vi "Make 16 to 8 LUT.vi"(1 "Black level":dbl format="%.2f", 2 "White level":dbl format="%.2f") -> (0 "Lookup Table":i16[](array[numeric]))   [LabVIEW 2011]
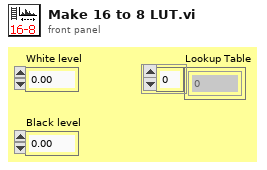
[diagram p1: front panel]
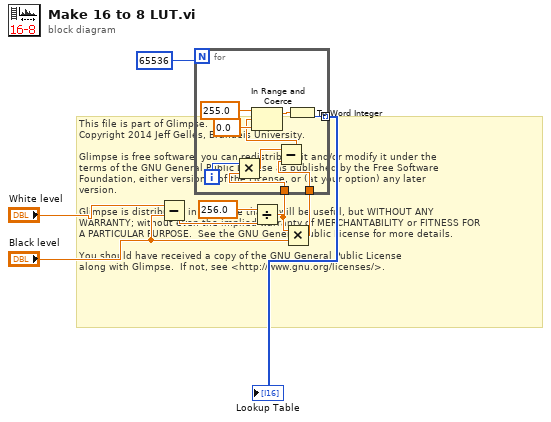
[diagram p0: block diagram]
diagram:
  # "This file is part of Glimpse. \nCopyright 2014 Jeff Gelles, Brandeis University.    \n\nGlimpse is free software: you can redistribute it and/or modify it under the \nterms of the GNU General Public License as published by the Free Software \nFoundation, either version 3 of the License, or (at your option) any later \nversion.\n\nGlimpse is distributed in the hope that it will be useful, but WITHOUT ANY \nWARRANTY; without even the implied warranty of MERCHANTABILITY or FITNESS FOR \nA PARTICULAR PURPOSE.  See the GNU General Public License for more details.\n\nYou should have received a copy of the GNU General Public License\nalong with Glimpse.  If not, see <http://www.gnu.org/licenses/>."
  n1 = Subtract(x="White level", y="Black level") -> (x-y=w3:dbl)
  n2 = Divide(x=256.0, y=w3) -> (x/y=w4:dbl)
  n3 = Multiply(x=w4, y="Black level") -> (x*y=w5:dbl)
  n4 = for {
    N: 65536 -> [_]
    tunnel: w4 -> [w16]
    tunnel: w5 -> [w15]
    tunnel: [w9] -> w8 mode=indexing
    i -> [w17]
    n5 = Multiply(x=w17, y=w16) -> (x*y=w14:dbl)
    n6 = Subtract(x=w14, y=w15) -> (x-y=w11:dbl)
    n7 = In Range and Coerce(upper limit=255.0, x=w11, lower limit=0.0) -> (coerced(x)=w10:dbl)  [unwired: 1 out]
    n8 = To Word Integer(number=w10) -> (16bit integer=w9:i16)
  }
  "Lookup Table" <- w8
